vi "example_subvi1.vi"(10 "y":dbl, 11 "Slide":dbl) -> (3 "Numeric":dbl)   [LabVIEW 2015]
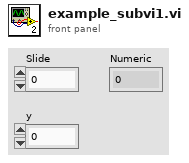
[diagram p1: front panel]
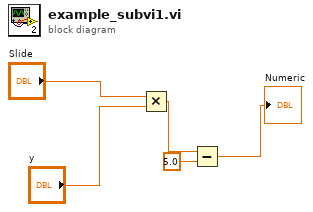
[diagram p0: block diagram]
diagram:
  n1 = Multiply(x="Slide", y="y") -> (x*y=w3:dbl)
  n2 = Subtract(x=w3, y=5.0) -> (x-y=→"Numeric":dbl)
